vi "Request Asynchronous Message.vi"(4 "Activate Immediately? (T)":bool=TRUE, 5 "Return Priority (Normal)":T2=enum."Normal", 6 "SubscriptionPolicy":refnum<class "ISubscriptionPolicy.lvclass">, 7 "Desired Notification Msg":refnum<class "Notification Msg.lvclass">, 8 "error in (no error)":errorcluster, 9 "Data Type":variant, 10 "Datum Name":string, 11 "IModel in":refnum<class "IModel.lvclass">) -> (0 "error out":errorcluster, 2 "Subscription Policy":T1, 3 "IModel out":refnum<class "IModel.lvclass">)   [LabVIEW 2017, in "IModel.lvlib" / "IModel.lvclass"]
doc: "DEPRECATED by IObserver.lvclass: Request Message.vi"
uses:
  IModel.lvclass
  C:/Program Files (x86)/National Instruments/LabVIEW 2017/vi.lib/ActorFramework/Actor/Actor.lvclass
  C:/Git/mva-framework/Source/Framework/IObserver/IObserver/IObserver.lvclass
  IMediator/ISubscriptionPolicy/ISubscriptionPolicy.lvclass
  gpm_packages/@cs/transport/Source/Concrete/ActorMessageTransport/Notification Msg/Notification Msg.lvclass
  <vilib>/ActorFramework/Message Enqueuer/Message Priority.ctl
  IMediator/ISubscriptionPolicy/ISubscriptionPolicy Reference.ctl
  IObserver/IObserver/IObserver.lvclass/IObserver.ctl
  <vilib>/ActorFramework/Actor/Actor.lvclass/Actor.ctl
  <vilib>/ActorFramework/Message Enqueuer/Message Enqueuer.lvclass/Message Enqueuer.ctl
  gpm_packages/@cs/transport/Source/Concrete/ActorMessageTransport/ActorMessageTransport.lvclass/ActorMessageTransport.ctl
  IMediator/SubscriptionRequest/SubscriptionRequest.lvclass/SubscriptionRequest.ctl
  AbstractMessages/PreAddressedMsg/PreAddressedMsg.lvclass/PreAddressedMsg.ctl
  IMediator/IMediator Messages/Subscribe Msg/Subscribe Msg.lvclass/Subscribe Msg.ctl
  <vilib>/ActorFramework/Message Enqueuer/Init from Existing Queue.vi
  <vilib>/ActorFramework/Message Enqueuer/Equals Not A Refnum.vi
  <vilib>/ActorFramework/Message Enqueuer/Enqueue.vi
  AbstractMessages/PreAddressedMsg/Read Return Address.vi
  gpm_packages/@cs/transport/Source/Concrete/ActorMessageTransport/ActorMessageTransport.lvclass
  C:/Git/mva-framework/gpm_packages/@cs/transport/Source/ITransport/ITransport.lvclass
  IMediator/IMediator Messages/Subscribe Msg/Subscribe Msg.lvclass
  C:/Git/mva-framework/Source/Framework/AbstractMessages/PreAddressedMsg/PreAddressedMsg.lvclass
  C:/Program Files (x86)/National Instruments/LabVIEW 2017/vi.lib/ActorFramework/Message/Message.lvclass
  <vilib>/Utility/error.llb/Error Cluster From Error Code.vi
  <vilib>/ActorFramework/Message Priority Queue/Priority Enqueue.vi
  <vilib>/ActorFramework/Message Enqueuer/Message Enqueuer.lvclass
  IMediator/SubscriptionRequest/SubscriptionRequest.lvclass
  <vilib>/ActorFramework/Actor/Actor.lvclass
  IObserver/IObserver/IObserver.lvclass
panel:
  # "Use IObserver.lvclass: Request Message.vi"
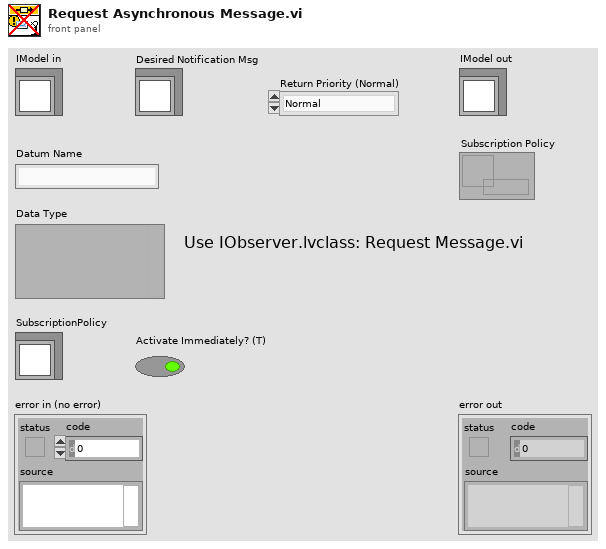
[diagram p1: front panel]
types:
  T1 = typedef "IMediator.lvlib/ISubscriptionPolicy.lvclass/ISubscriptionPolicy Reference.ctl" = refnum<data-value>
  T2 = typedef "Actor Framework.lvlib/Message Enqueuer.lvclass/Message Priority.ctl" = enum16{"Low", "Normal", "High"}
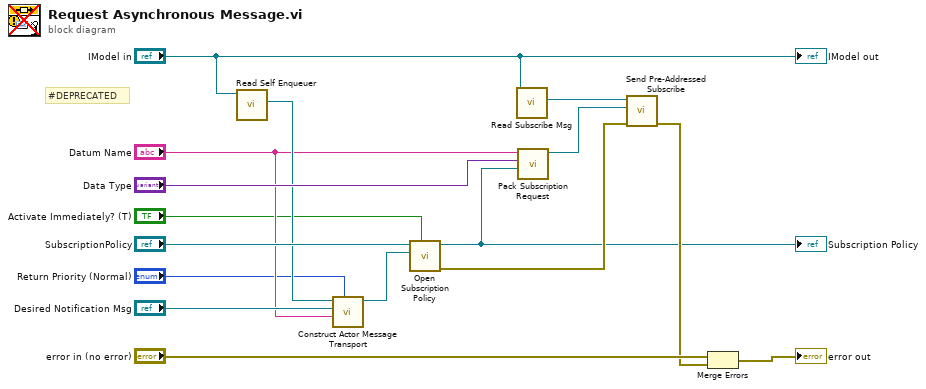
[diagram p0: block diagram]
diagram:
  # "#DEPRECATED"
  n1 = call <vilib>:"Read Self Enqueuer.vi"("Actor"="IModel in") -> ("Self Enqueuer"=w7:refnum<class "Message Enqueuer.lvclass">)  [unwired: 10 in]
  n2 = call "Construct Actor Message Transport.vi"("Return Priority (Normal)"="Return Priority (Normal)", "Datum Name"="Datum Name", "Notification Msg"="Desired Notification Msg", "Message Enqueuer in"=w7) -> ("ActorMessageTransport"=w14:refnum<class "ActorMessageTransport.lvclass">)  [unwired: 6 in, 1 out]
  n3 = call "Open Subscription Policy.vi"("Activate? (T)"="Activate Immediately? (T)", "Transport"=w14, "SubscriptionPolicy"="SubscriptionPolicy") -> ("error out"=w10:errorcluster, "Subscription Policy"=w2:T1)  [unwired: 7 in]
  "Subscription Policy" <- w2
  n4 = call "Read Subscribe Msg.vi"("IObserver in"="IModel in") -> ("Pre-Addressed Subscribe Msg"=w13:refnum<class "Subscribe Msg.lvclass">)  [unwired: 10 in]
  n5 = call "Pack Subscription Request.vi"("Subscription Policy"=w2, "Type"="Data Type", "Datum Name"="Datum Name") -> ("SubscriptionRequest"=w12:refnum<class "SubscriptionRequest.lvclass">)  [unwired: 8 in]
  n6 = call "Send Pre-Addressed Subscribe.vi"("error in (no error)"=w10, "Subscription Request"=w12, "Subscribe Msg"=w13) -> ("error out"=w8:errorcluster)  [unwired: 8 in]
  n7 = Merge Errors("error in (no error)", w8) -> (→"error out":errorcluster)
  "IModel out" <- "IModel in"
